vi "_Main.vi"   [LabVIEW 2016, in "TemplateSensor.lvlib"]
uses:
  TemplateSensor.lvlib
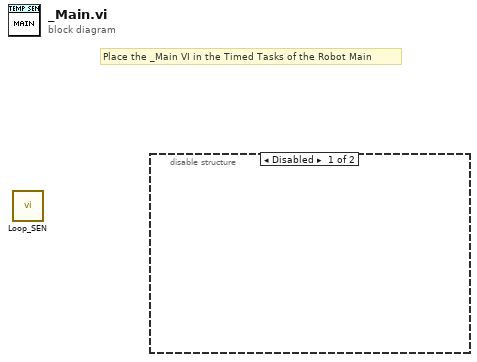
[diagram p0: block diagram]
diagram:
  # "Place the _Main VI in the Timed Tasks of the Robot Main"
  n1 = call "Loop_SEN.vi"() -> ()  [unwired: 12 in]
  n2 = disable-structure shown="Disabled" {
    frame Disabled {
    }
    frame Enabled {
    }
  }
